vi "Run - Array of Status Monitors With Transient Captures.vi"() -> ()   [LabVIEW 2017]
uses:
  Communications/Communications Library.lvlib
panel:
  in  "configuration file path":path
  in  "Pre-Trigger Samples":i32
  in  "Post-Trigger Samples":i32=100000
  in  "Soft Trigger":bool
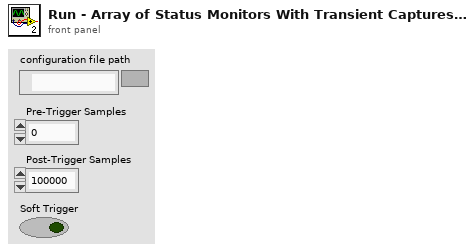
[diagram p1: front panel]
types:
  T1 = enum32{"Invalid", "Standard", "Closed", "Hidden", "Minimized", "Maximized"}
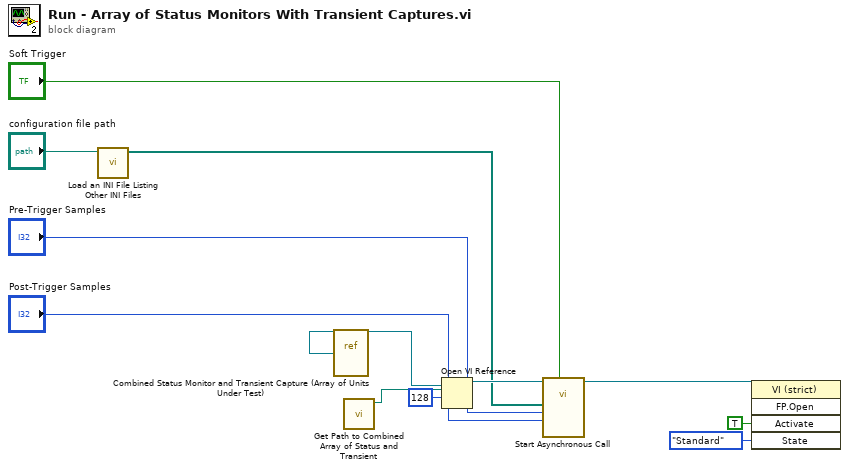
[diagram p0: block diagram]
diagram:
  n1 = call "Load an INI File Listing Other INI Files.vi"("configuration file path"="configuration file path") -> ("Array"=w2:path[])  [unwired: 9 in, 1 out]
  n2 = vi-ref "Combined Status Monitor and Transient Capture (Array of Units Under Test).vi"() -> (w12:refnum<vi>)
  n3 = call "Get Path to Combined Array of Status and Transient.vi"() -> ("Path to Combined Status and Transient"=w11:path)  [unwired: 11 in]
  n4 = Open VI Reference(type specifier VI Refnum (for type only)=w12, vi path=w11, options=128) -> (vi reference=w9:refnum<vi>)  [unwired: 3 in, 1 out]
  n5 = call-by-ref "Start Asynchronous Call"(reference=w9, "Soft Trigger"="Soft Trigger", "Post-Trigger Samples"="Post-Trigger Samples", "Pre-Trigger Samples"="Pre-Trigger Samples", "List of INI Files"=w2) -> (reference out=w5:refnum<vi>)  [unwired: 9 in, 1 out]
  n6 = invoke class="VI (strict)" method="FP.Open"(reference=w5, "Activate"=TRUE ("Activate?"), "State"=T1."Standard") -> ()  [unwired: 2 in, 5 out]
